vi "decodeArray.vi"(8 "error in (no error)":errorcluster, 9 "Map to Cluster?(T)":bool, 11 "ByteArray":u8[](array[numeric]) format="%x") -> (0 "error out":errorcluster, 2 "Variant":variant, 3 "RemainingBytes":u8[](array[numeric]) format="%x", 5 "Type":string)   [LabVIEW 2015, in "MsgPack.lvlib"]
uses:
  MsgPack.lvlib
panel:
  out "Array":string[](array[string])
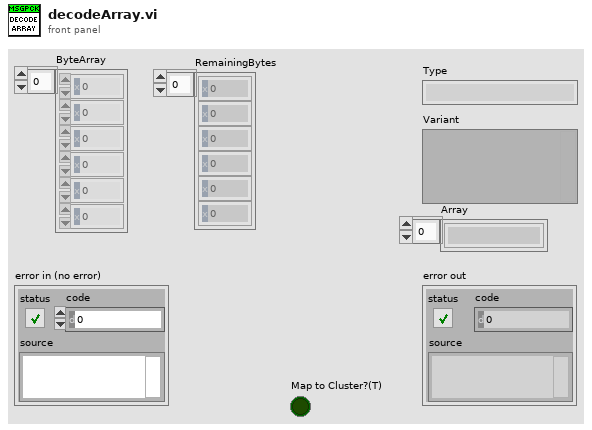
[diagram p1: front panel]
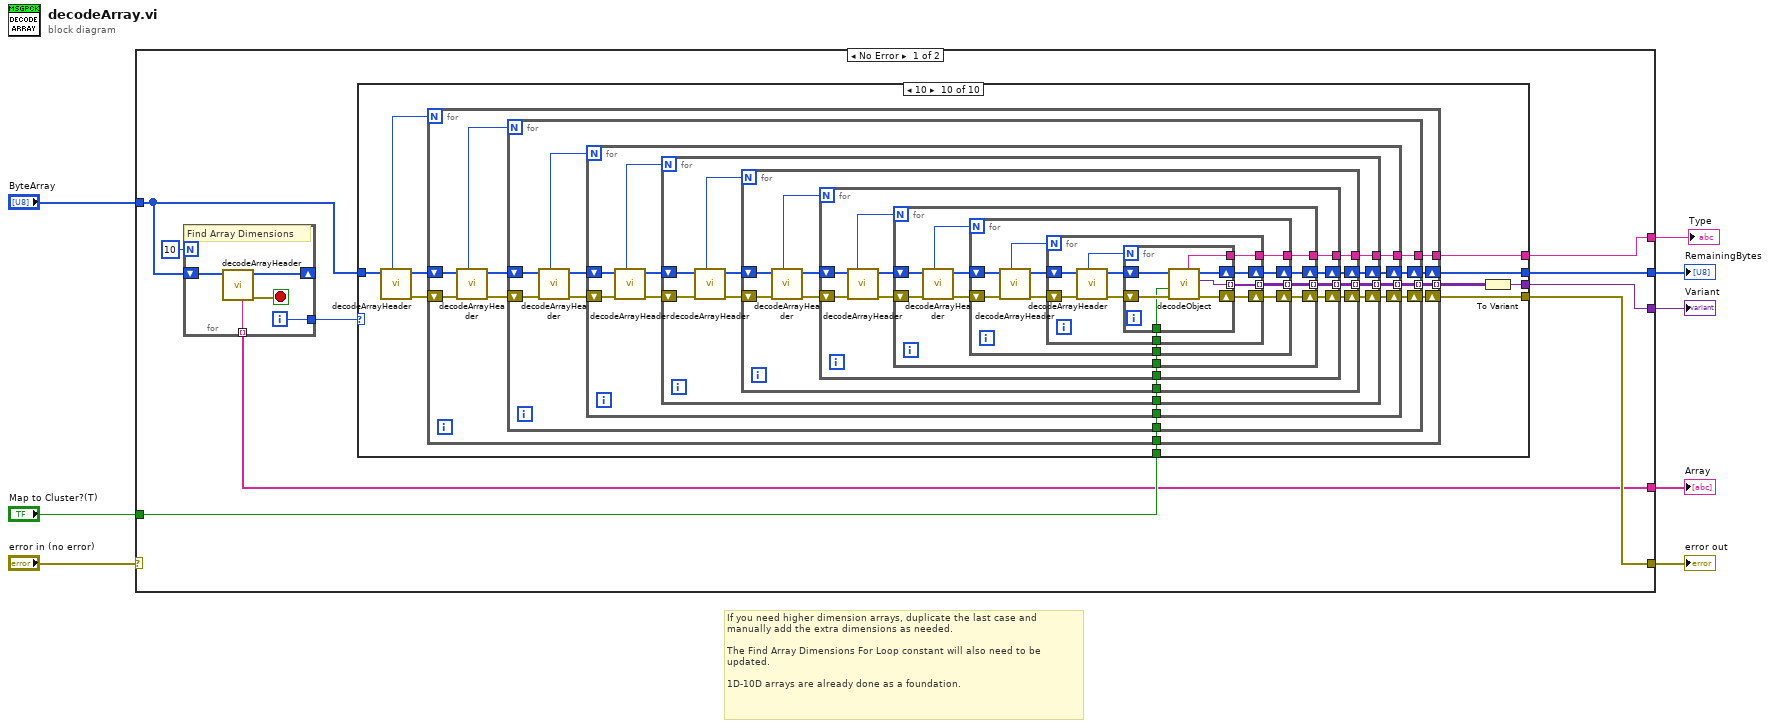
[diagram p0: block diagram]
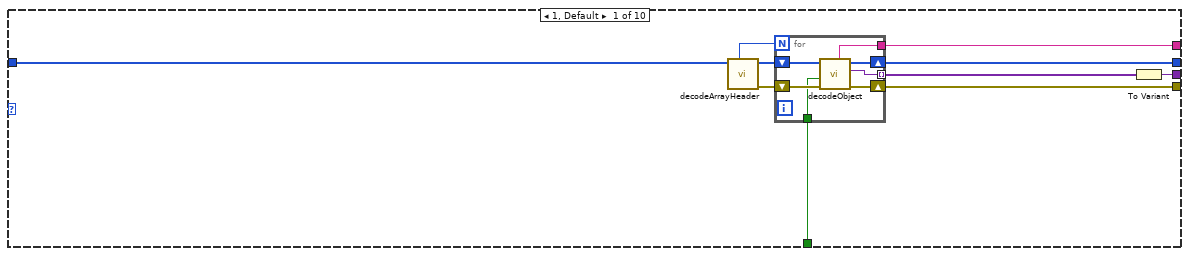
[diagram p2: hidden frame]
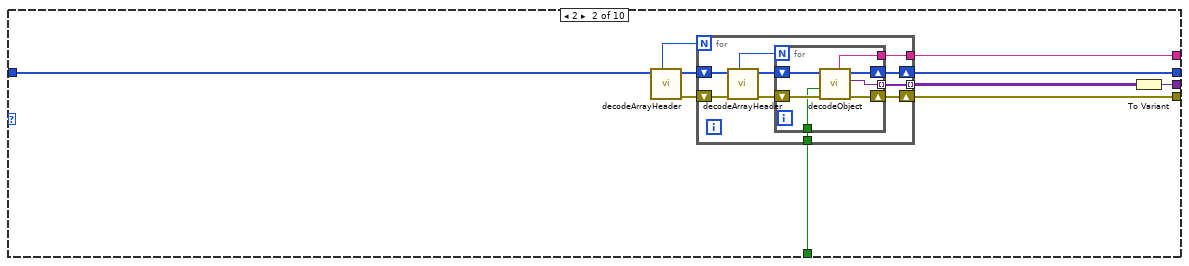
[diagram p3: hidden frame]
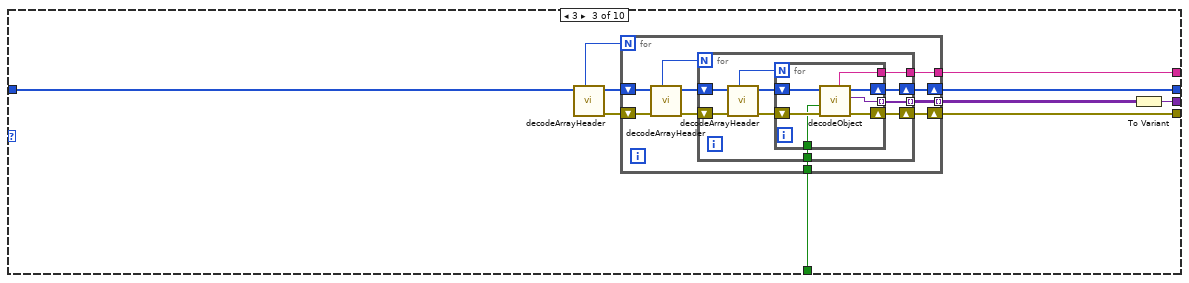
[diagram p4: hidden frame]
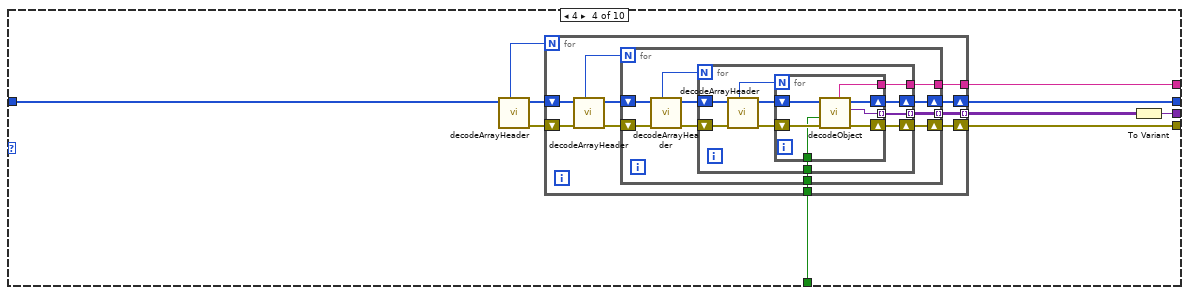
[diagram p5: hidden frame]
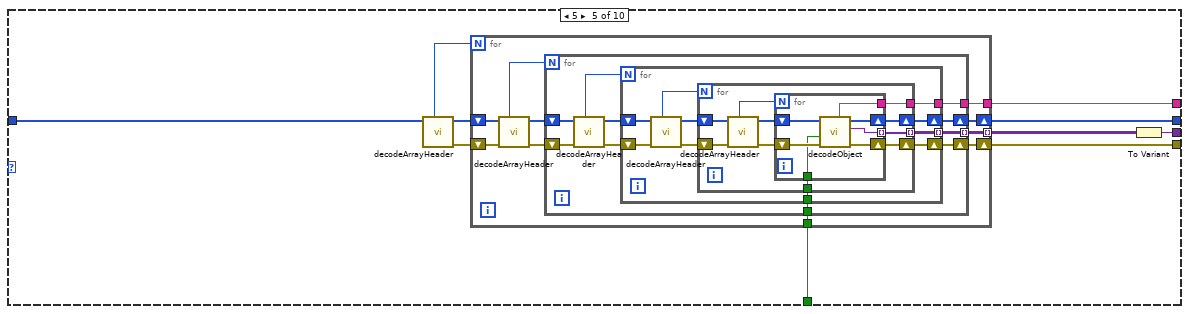
[diagram p6: hidden frame]
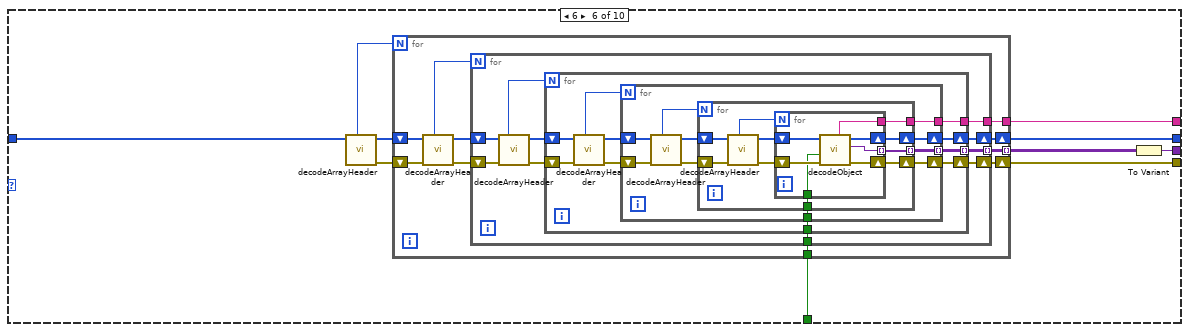
[diagram p7: hidden frame]
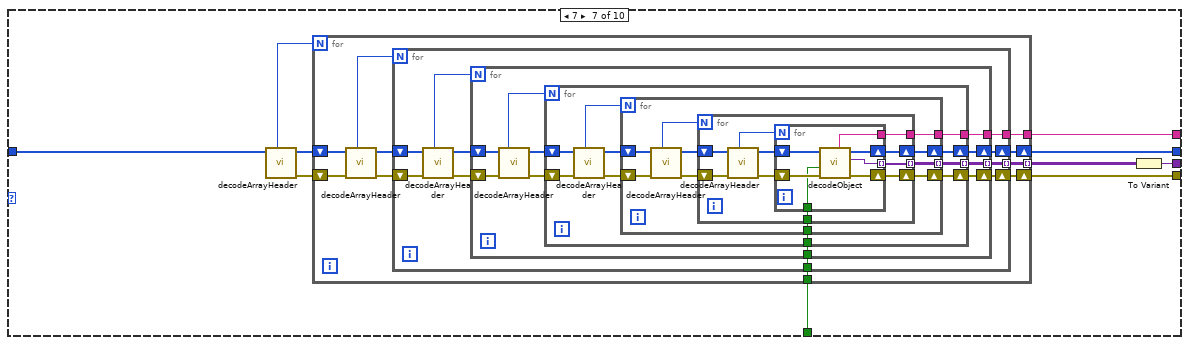
[diagram p8: hidden frame]
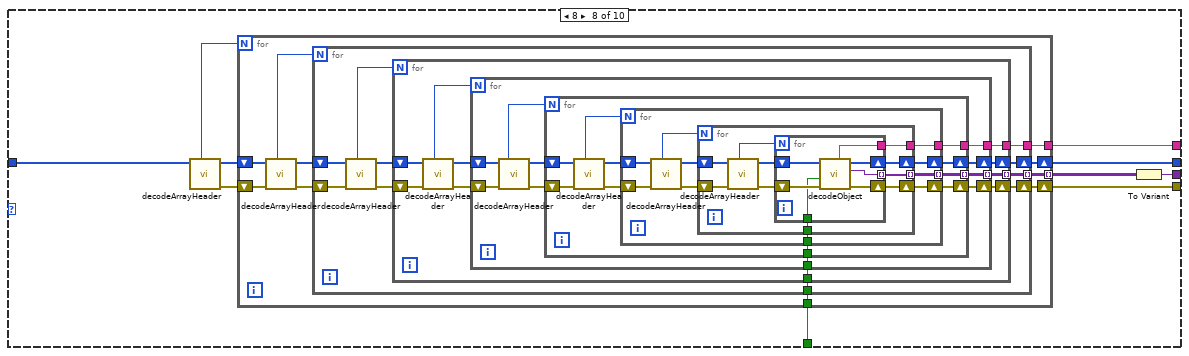
[diagram p9: hidden frame]
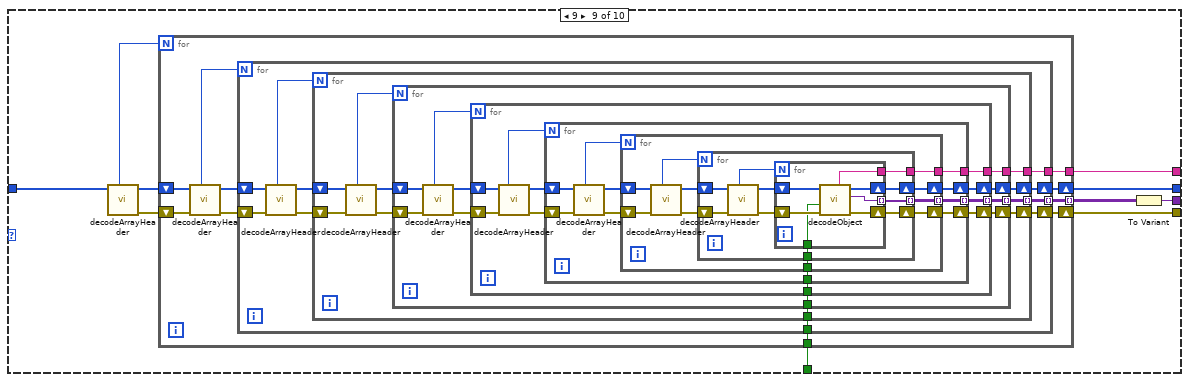
[diagram p10: hidden frame]
diagram:
  # "If you need higher dimension arrays, duplicate the last case and manually add the extra dimensions as needed.\n\nThe Find Array Dimensions For Loop constant will also need to be updated.\n\n1D-10D arrays are already done as a foundation."
  n1 = case shown="No Error" "error in (no error)" {
    selector: "error in (no error)" -> [_ w644]
    tunnel: [w17 w644] -> w8
    tunnel: "ByteArray" -> [w13 w643]
    tunnel: [w16 w643] -> w6
    tunnel: [w12 _] -> w4
    tunnel: [w11 _] -> w3
    tunnel: [w10 _] -> w2
    tunnel: "Map to Cluster?(T)" -> [w15 _]
    frame No Error {
      n2 = for {
        N: 10 -> [_]
        shift-right: [w641] -> _
        shift-left: w13 -> [w642]
        tunnel: [w639] -> w14
        tunnel: [w638] -> w11 mode=indexing
        i -> [w639]
        stop <- w640 stop-if-true
        # "Find Array Dimensions"
        n3 = call "decodeArrayHeader.vi"("ByteArray"=w642) -> ("error out"=w640:errorcluster, "RemainingBytes"=w641:u8[], "Type"=w638:string)  [unwired: 7 in, 1 out]
      }
      n4 = case shown="10" w14 {
        tunnel: [w27 w44 w71 w108 w155 w212 w279 w356 w443 w540] -> w17
        tunnel: [w26 w43 w70 w107 w154 w211 w278 w355 w442 w539] -> w16
        tunnel: w15 -> [w22 w42 w69 w106 w153 w210 w277 w354 w441 w538]
        tunnel: w13 -> [w21 w38 w65 w100 w148 w206 w271 w347 w437 w534]
        tunnel: [w19 w40 w67 w104 w151 w208 w275 w352 w439 w536] -> w12
        tunnel: [w18 w39 w66 w103 w150 w207 w274 w351 w438 w535] -> w10
        frame 1, Default {
          n5 = call "decodeArrayHeader.vi"("ByteArray"=w21) -> ("error out"=w24:errorcluster, "RemainingBytes"=w25:u8[], "Array Size"=w23:u32)  [unwired: 7 in, 1 out]
          n6 = for {
            N: w23 -> [_]
            shift-right: [w32] -> w26
            shift-left: w25 -> [w33]
            shift-right: [w30] -> w27
            shift-left: w24 -> [w34]
            tunnel: [w31] -> w20 mode=indexing
            tunnel: w22 -> [w29]
            tunnel: [w28] -> w18
            n7 = call "decodeObject.vi"("error in (no error)"=w34, "Map to Cluster?(T)"=w29, "ByteArray"=w33) -> ("error out"=w30:errorcluster, "Variant"=w31:variant, "RemainingBytes"=w32:u8[], "Type"=w28:string)  [unwired: 5 in]
          }
          n8 = To Variant(anything=w20) -> (Variant=w19:variant)
        }
        frame 2 {
          n9 = call "decodeArrayHeader.vi"("ByteArray"=w38) -> ("error out"=w36:errorcluster, "RemainingBytes"=w37:u8[], "Array Size"=w35:u32)  [unwired: 7 in, 1 out]
          n10 = for {
            N: w35 -> [_]
            tunnel: w42 -> [w49]
            tunnel: [w47] -> w41 mode=indexing
            tunnel: [w46] -> w39
            shift-right: [w53] -> w43
            shift-left: w37 -> [w48]
            shift-right: [w54] -> w44
            shift-left: w36 -> [w45]
            n11 = call "decodeArrayHeader.vi"("error in (no error)"=w45, "ByteArray"=w48) -> ("error out"=w51:errorcluster, "RemainingBytes"=w52:u8[], "Array Size"=w50:u32)  [unwired: 6 in, 1 out]
            n12 = for {
              N: w50 -> [_]
              shift-right: [w59] -> w53
              shift-left: w52 -> [w60]
              shift-right: [w57] -> w54
              shift-left: w51 -> [w61]
              tunnel: [w58] -> w47 mode=indexing
              tunnel: w49 -> [w56]
              tunnel: [w55] -> w46
              n13 = call "decodeObject.vi"("error in (no error)"=w61, "Map to Cluster?(T)"=w56, "ByteArray"=w60) -> ("error out"=w57:errorcluster, "Variant"=w58:variant, "RemainingBytes"=w59:u8[], "Type"=w55:string)  [unwired: 5 in]
            }
          }
          n14 = To Variant(anything=w41) -> (Variant=w40:variant)
        }
        frame 3 {
          n15 = call "decodeArrayHeader.vi"("ByteArray"=w65) -> ("error out"=w63:errorcluster, "RemainingBytes"=w64:u8[], "Array Size"=w62:u32)  [unwired: 7 in, 1 out]
          n16 = for {
            N: w62 -> [_]
            tunnel: w69 -> [w79]
            tunnel: [w78] -> w68 mode=indexing
            tunnel: [w77] -> w66
            shift-right: [w80] -> w70
            shift-left: w64 -> [w76]
            shift-right: [w81] -> w71
            shift-left: w63 -> [w72]
            n17 = call "decodeArrayHeader.vi"("error in (no error)"=w72, "ByteArray"=w76) -> ("error out"=w74:errorcluster, "RemainingBytes"=w75:u8[], "Array Size"=w73:u32)  [unwired: 6 in, 1 out]
            n18 = for {
              N: w73 -> [_]
              tunnel: w79 -> [w86]
              tunnel: [w84] -> w78 mode=indexing
              tunnel: [w83] -> w77
              shift-right: [w90] -> w80
              shift-left: w75 -> [w85]
              shift-right: [w91] -> w81
              shift-left: w74 -> [w82]
              n19 = call "decodeArrayHeader.vi"("error in (no error)"=w82, "ByteArray"=w85) -> ("error out"=w88:errorcluster, "RemainingBytes"=w89:u8[], "Array Size"=w87:u32)  [unwired: 6 in, 1 out]
              n20 = for {
                N: w87 -> [_]
                shift-right: [w96] -> w90
                shift-left: w89 -> [w97]
                shift-right: [w94] -> w91
                shift-left: w88 -> [w98]
                tunnel: [w95] -> w84 mode=indexing
                tunnel: w86 -> [w93]
                tunnel: [w92] -> w83
                n21 = call "decodeObject.vi"("error in (no error)"=w98, "Map to Cluster?(T)"=w93, "ByteArray"=w97) -> ("error out"=w94:errorcluster, "Variant"=w95:variant, "RemainingBytes"=w96:u8[], "Type"=w92:string)  [unwired: 5 in]
              }
            }
          }
          n22 = To Variant(anything=w68) -> (Variant=w67:variant)
        }
        frame 4 {
          n23 = call "decodeArrayHeader.vi"("ByteArray"=w100) -> ("error out"=w102:errorcluster, "RemainingBytes"=w101:u8[], "Array Size"=w99:u32)  [unwired: 7 in, 1 out]
          n24 = for {
            N: w99 -> [_]
            tunnel: w106 -> [w116]
            tunnel: [w115] -> w105 mode=indexing
            tunnel: [w114] -> w103
            shift-right: [w117] -> w107
            shift-left: w101 -> [w113]
            shift-right: [w118] -> w108
            shift-left: w102 -> [w109]
            n25 = call "decodeArrayHeader.vi"("error in (no error)"=w109, "ByteArray"=w113) -> ("error out"=w111:errorcluster, "RemainingBytes"=w112:u8[], "Array Size"=w110:u32)  [unwired: 6 in, 1 out]
            n26 = for {
              N: w110 -> [_]
              tunnel: w116 -> [w126]
              tunnel: [w125] -> w115 mode=indexing
              tunnel: [w124] -> w114
              shift-right: [w127] -> w117
              shift-left: w112 -> [w123]
              shift-right: [w128] -> w118
              shift-left: w111 -> [w119]
              n27 = call "decodeArrayHeader.vi"("error in (no error)"=w119, "ByteArray"=w123) -> ("error out"=w121:errorcluster, "RemainingBytes"=w122:u8[], "Array Size"=w120:u32)  [unwired: 6 in, 1 out]
              n28 = for {
                N: w120 -> [_]
                tunnel: w126 -> [w133]
                tunnel: [w131] -> w125 mode=indexing
                tunnel: [w130] -> w124
                shift-right: [w137] -> w127
                shift-left: w122 -> [w132]
                shift-right: [w138] -> w128
                shift-left: w121 -> [w129]
                n29 = call "decodeArrayHeader.vi"("error in (no error)"=w129, "ByteArray"=w132) -> ("error out"=w135:errorcluster, "RemainingBytes"=w136:u8[], "Array Size"=w134:u32)  [unwired: 6 in, 1 out]
                n30 = for {
                  N: w134 -> [_]
                  shift-right: [w143] -> w137
                  shift-left: w136 -> [w144]
                  shift-right: [w141] -> w138
                  shift-left: w135 -> [w145]
                  tunnel: [w142] -> w131 mode=indexing
                  tunnel: w133 -> [w140]
                  tunnel: [w139] -> w130
                  n31 = call "decodeObject.vi"("error in (no error)"=w145, "Map to Cluster?(T)"=w140, "ByteArray"=w144) -> ("error out"=w141:errorcluster, "Variant"=w142:variant, "RemainingBytes"=w143:u8[], "Type"=w139:string)  [unwired: 5 in]
                }
              }
            }
          }
          n32 = To Variant(anything=w105) -> (Variant=w104:variant)
        }
        frame 5 {
          n33 = call "decodeArrayHeader.vi"("ByteArray"=w148) -> ("error out"=w149:errorcluster, "RemainingBytes"=w147:u8[], "Array Size"=w146:u32)  [unwired: 7 in, 1 out]
          n34 = for {
            N: w146 -> [_]
            tunnel: w153 -> [w163]
            tunnel: [w162] -> w152 mode=indexing
            tunnel: [w161] -> w150
            shift-right: [w164] -> w154
            shift-left: w147 -> [w158]
            shift-right: [w165] -> w155
            shift-left: w149 -> [w157]
            n35 = call "decodeArrayHeader.vi"("error in (no error)"=w157, "ByteArray"=w158) -> ("error out"=w160:errorcluster, "RemainingBytes"=w159:u8[], "Array Size"=w156:u32)  [unwired: 6 in, 1 out]
            n36 = for {
              N: w156 -> [_]
              tunnel: w163 -> [w173]
              tunnel: [w172] -> w162 mode=indexing
              tunnel: [w171] -> w161
              shift-right: [w174] -> w164
              shift-left: w159 -> [w170]
              shift-right: [w175] -> w165
              shift-left: w160 -> [w166]
              n37 = call "decodeArrayHeader.vi"("error in (no error)"=w166, "ByteArray"=w170) -> ("error out"=w168:errorcluster, "RemainingBytes"=w169:u8[], "Array Size"=w167:u32)  [unwired: 6 in, 1 out]
              n38 = for {
                N: w167 -> [_]
                tunnel: w173 -> [w183]
                tunnel: [w182] -> w172 mode=indexing
                tunnel: [w181] -> w171
                shift-right: [w184] -> w174
                shift-left: w169 -> [w180]
                shift-right: [w185] -> w175
                shift-left: w168 -> [w176]
                n39 = call "decodeArrayHeader.vi"("error in (no error)"=w176, "ByteArray"=w180) -> ("error out"=w178:errorcluster, "RemainingBytes"=w179:u8[], "Array Size"=w177:u32)  [unwired: 6 in, 1 out]
                n40 = for {
                  N: w177 -> [_]
                  tunnel: w183 -> [w190]
                  tunnel: [w188] -> w182 mode=indexing
                  tunnel: [w187] -> w181
                  shift-right: [w194] -> w184
                  shift-left: w179 -> [w189]
                  shift-right: [w195] -> w185
                  shift-left: w178 -> [w186]
                  n41 = call "decodeArrayHeader.vi"("error in (no error)"=w186, "ByteArray"=w189) -> ("error out"=w192:errorcluster, "RemainingBytes"=w193:u8[], "Array Size"=w191:u32)  [unwired: 6 in, 1 out]
                  n42 = for {
                    N: w191 -> [_]
                    shift-right: [w200] -> w194
                    shift-left: w193 -> [w201]
                    shift-right: [w198] -> w195
                    shift-left: w192 -> [w202]
                    tunnel: [w199] -> w188 mode=indexing
                    tunnel: w190 -> [w197]
                    tunnel: [w196] -> w187
                    n43 = call "decodeObject.vi"("error in (no error)"=w202, "Map to Cluster?(T)"=w197, "ByteArray"=w201) -> ("error out"=w198:errorcluster, "Variant"=w199:variant, "RemainingBytes"=w200:u8[], "Type"=w196:string)  [unwired: 5 in]
                  }
                }
              }
            }
          }
          n44 = To Variant(anything=w152) -> (Variant=w151:variant)
        }
        frame 6 {
          n45 = call "decodeArrayHeader.vi"("ByteArray"=w206) -> ("error out"=w205:errorcluster, "RemainingBytes"=w204:u8[], "Array Size"=w203:u32)  [unwired: 7 in, 1 out]
          n46 = for {
            N: w203 -> [_]
            tunnel: w210 -> [w220]
            tunnel: [w219] -> w209 mode=indexing
            tunnel: [w218] -> w207
            shift-right: [w221] -> w211
            shift-left: w204 -> [w216]
            shift-right: [w222] -> w212
            shift-left: w205 -> [w214]
            n47 = call "decodeArrayHeader.vi"("error in (no error)"=w214, "ByteArray"=w216) -> ("error out"=w217:errorcluster, "RemainingBytes"=w215:u8[], "Array Size"=w213:u32)  [unwired: 6 in, 1 out]
            n48 = for {
              N: w213 -> [_]
              tunnel: w220 -> [w230]
              tunnel: [w229] -> w219 mode=indexing
              tunnel: [w228] -> w218
              shift-right: [w231] -> w221
              shift-left: w215 -> [w225]
              shift-right: [w232] -> w222
              shift-left: w217 -> [w224]
              n49 = call "decodeArrayHeader.vi"("error in (no error)"=w224, "ByteArray"=w225) -> ("error out"=w227:errorcluster, "RemainingBytes"=w226:u8[], "Array Size"=w223:u32)  [unwired: 6 in, 1 out]
              n50 = for {
                N: w223 -> [_]
                tunnel: w230 -> [w240]
                tunnel: [w239] -> w229 mode=indexing
                tunnel: [w238] -> w228
                shift-right: [w241] -> w231
                shift-left: w226 -> [w237]
                shift-right: [w242] -> w232
                shift-left: w227 -> [w233]
                n51 = call "decodeArrayHeader.vi"("error in (no error)"=w233, "ByteArray"=w237) -> ("error out"=w235:errorcluster, "RemainingBytes"=w236:u8[], "Array Size"=w234:u32)  [unwired: 6 in, 1 out]
                n52 = for {
                  N: w234 -> [_]
                  tunnel: w240 -> [w250]
                  tunnel: [w249] -> w239 mode=indexing
                  tunnel: [w248] -> w238
                  shift-right: [w251] -> w241
                  shift-left: w236 -> [w247]
                  shift-right: [w252] -> w242
                  shift-left: w235 -> [w243]
                  n53 = call "decodeArrayHeader.vi"("error in (no error)"=w243, "ByteArray"=w247) -> ("error out"=w245:errorcluster, "RemainingBytes"=w246:u8[], "Array Size"=w244:u32)  [unwired: 6 in, 1 out]
                  n54 = for {
                    N: w244 -> [_]
                    tunnel: w250 -> [w257]
                    tunnel: [w255] -> w249 mode=indexing
                    tunnel: [w254] -> w248
                    shift-right: [w261] -> w251
                    shift-left: w246 -> [w256]
                    shift-right: [w262] -> w252
                    shift-left: w245 -> [w253]
                    n55 = call "decodeArrayHeader.vi"("error in (no error)"=w253, "ByteArray"=w256) -> ("error out"=w259:errorcluster, "RemainingBytes"=w260:u8[], "Array Size"=w258:u32)  [unwired: 6 in, 1 out]
                    n56 = for {
                      N: w258 -> [_]
                      shift-right: [w267] -> w261
                      shift-left: w260 -> [w268]
                      shift-right: [w265] -> w262
                      shift-left: w259 -> [w269]
                      tunnel: [w266] -> w255 mode=indexing
                      tunnel: w257 -> [w264]
                      tunnel: [w263] -> w254
                      n57 = call "decodeObject.vi"("error in (no error)"=w269, "Map to Cluster?(T)"=w264, "ByteArray"=w268) -> ("error out"=w265:errorcluster, "Variant"=w266:variant, "RemainingBytes"=w267:u8[], "Type"=w263:string)  [unwired: 5 in]
                    }
                  }
                }
              }
            }
          }
          n58 = To Variant(anything=w209) -> (Variant=w208:variant)
        }
        frame 7 {
          n59 = call "decodeArrayHeader.vi"("ByteArray"=w271) -> ("error out"=w273:errorcluster, "RemainingBytes"=w272:u8[], "Array Size"=w270:u32)  [unwired: 7 in, 1 out]
          n60 = for {
            N: w270 -> [_]
            tunnel: w277 -> [w287]
            tunnel: [w286] -> w276 mode=indexing
            tunnel: [w285] -> w274
            shift-right: [w288] -> w278
            shift-left: w272 -> [w284]
            shift-right: [w289] -> w279
            shift-left: w273 -> [w280]
            n61 = call "decodeArrayHeader.vi"("error in (no error)"=w280, "ByteArray"=w284) -> ("error out"=w283:errorcluster, "RemainingBytes"=w282:u8[], "Array Size"=w281:u32)  [unwired: 6 in, 1 out]
            n62 = for {
              N: w281 -> [_]
              tunnel: w287 -> [w297]
              tunnel: [w296] -> w286 mode=indexing
              tunnel: [w295] -> w285
              shift-right: [w298] -> w288
              shift-left: w282 -> [w293]
              shift-right: [w299] -> w289
              shift-left: w283 -> [w291]
              n63 = call "decodeArrayHeader.vi"("error in (no error)"=w291, "ByteArray"=w293) -> ("error out"=w294:errorcluster, "RemainingBytes"=w292:u8[], "Array Size"=w290:u32)  [unwired: 6 in, 1 out]
              n64 = for {
                N: w290 -> [_]
                tunnel: w297 -> [w307]
                tunnel: [w306] -> w296 mode=indexing
                tunnel: [w305] -> w295
                shift-right: [w308] -> w298
                shift-left: w292 -> [w302]
                shift-right: [w309] -> w299
                shift-left: w294 -> [w301]
                n65 = call "decodeArrayHeader.vi"("error in (no error)"=w301, "ByteArray"=w302) -> ("error out"=w304:errorcluster, "RemainingBytes"=w303:u8[], "Array Size"=w300:u32)  [unwired: 6 in, 1 out]
                n66 = for {
                  N: w300 -> [_]
                  tunnel: w307 -> [w317]
                  tunnel: [w316] -> w306 mode=indexing
                  tunnel: [w315] -> w305
                  shift-right: [w318] -> w308
                  shift-left: w303 -> [w314]
                  shift-right: [w319] -> w309
                  shift-left: w304 -> [w310]
                  n67 = call "decodeArrayHeader.vi"("error in (no error)"=w310, "ByteArray"=w314) -> ("error out"=w312:errorcluster, "RemainingBytes"=w313:u8[], "Array Size"=w311:u32)  [unwired: 6 in, 1 out]
                  n68 = for {
                    N: w311 -> [_]
                    tunnel: w317 -> [w327]
                    tunnel: [w326] -> w316 mode=indexing
                    tunnel: [w325] -> w315
                    shift-right: [w328] -> w318
                    shift-left: w313 -> [w324]
                    shift-right: [w329] -> w319
                    shift-left: w312 -> [w320]
                    n69 = call "decodeArrayHeader.vi"("error in (no error)"=w320, "ByteArray"=w324) -> ("error out"=w322:errorcluster, "RemainingBytes"=w323:u8[], "Array Size"=w321:u32)  [unwired: 6 in, 1 out]
                    n70 = for {
                      N: w321 -> [_]
                      tunnel: w327 -> [w334]
                      tunnel: [w332] -> w326 mode=indexing
                      tunnel: [w331] -> w325
                      shift-right: [w338] -> w328
                      shift-left: w323 -> [w333]
                      shift-right: [w339] -> w329
                      shift-left: w322 -> [w330]
                      n71 = call "decodeArrayHeader.vi"("error in (no error)"=w330, "ByteArray"=w333) -> ("error out"=w336:errorcluster, "RemainingBytes"=w337:u8[], "Array Size"=w335:u32)  [unwired: 6 in, 1 out]
                      n72 = for {
                        N: w335 -> [_]
                        shift-right: [w344] -> w338
                        shift-left: w337 -> [w345]
                        shift-right: [w342] -> w339
                        shift-left: w336 -> [w346]
                        tunnel: [w343] -> w332 mode=indexing
                        tunnel: w334 -> [w341]
                        tunnel: [w340] -> w331
                        n73 = call "decodeObject.vi"("error in (no error)"=w346, "Map to Cluster?(T)"=w341, "ByteArray"=w345) -> ("error out"=w342:errorcluster, "Variant"=w343:variant, "RemainingBytes"=w344:u8[], "Type"=w340:string)  [unwired: 5 in]
                      }
                    }
                  }
                }
              }
            }
          }
          n74 = To Variant(anything=w276) -> (Variant=w275:variant)
        }
        frame 8 {
          n75 = call "decodeArrayHeader.vi"("ByteArray"=w347) -> ("error out"=w349:errorcluster, "RemainingBytes"=w350:u8[], "Array Size"=w348:u32)  [unwired: 7 in, 1 out]
          n76 = for {
            N: w348 -> [_]
            tunnel: w354 -> [w364]
            tunnel: [w363] -> w353 mode=indexing
            tunnel: [w362] -> w351
            shift-right: [w365] -> w355
            shift-left: w350 -> [w359]
            shift-right: [w366] -> w356
            shift-left: w349 -> [w357]
            n77 = call "decodeArrayHeader.vi"("error in (no error)"=w357, "ByteArray"=w359) -> ("error out"=w361:errorcluster, "RemainingBytes"=w360:u8[], "Array Size"=w358:u32)  [unwired: 6 in, 1 out]
            n78 = for {
              N: w358 -> [_]
              tunnel: w364 -> [w374]
              tunnel: [w373] -> w363 mode=indexing
              tunnel: [w372] -> w362
              shift-right: [w375] -> w365
              shift-left: w360 -> [w371]
              shift-right: [w376] -> w366
              shift-left: w361 -> [w367]
              n79 = call "decodeArrayHeader.vi"("error in (no error)"=w367, "ByteArray"=w371) -> ("error out"=w370:errorcluster, "RemainingBytes"=w369:u8[], "Array Size"=w368:u32)  [unwired: 6 in, 1 out]
              n80 = for {
                N: w368 -> [_]
                tunnel: w374 -> [w384]
                tunnel: [w383] -> w373 mode=indexing
                tunnel: [w382] -> w372
                shift-right: [w385] -> w375
                shift-left: w369 -> [w380]
                shift-right: [w386] -> w376
                shift-left: w370 -> [w378]
                n81 = call "decodeArrayHeader.vi"("error in (no error)"=w378, "ByteArray"=w380) -> ("error out"=w381:errorcluster, "RemainingBytes"=w379:u8[], "Array Size"=w377:u32)  [unwired: 6 in, 1 out]
                n82 = for {
                  N: w377 -> [_]
                  tunnel: w384 -> [w394]
                  tunnel: [w393] -> w383 mode=indexing
                  tunnel: [w392] -> w382
                  shift-right: [w395] -> w385
                  shift-left: w379 -> [w389]
                  shift-right: [w396] -> w386
                  shift-left: w381 -> [w388]
                  n83 = call "decodeArrayHeader.vi"("error in (no error)"=w388, "ByteArray"=w389) -> ("error out"=w391:errorcluster, "RemainingBytes"=w390:u8[], "Array Size"=w387:u32)  [unwired: 6 in, 1 out]
                  n84 = for {
                    N: w387 -> [_]
                    tunnel: w394 -> [w404]
                    tunnel: [w403] -> w393 mode=indexing
                    tunnel: [w402] -> w392
                    shift-right: [w405] -> w395
                    shift-left: w390 -> [w401]
                    shift-right: [w406] -> w396
                    shift-left: w391 -> [w397]
                    n85 = call "decodeArrayHeader.vi"("error in (no error)"=w397, "ByteArray"=w401) -> ("error out"=w399:errorcluster, "RemainingBytes"=w400:u8[], "Array Size"=w398:u32)  [unwired: 6 in, 1 out]
                    n86 = for {
                      N: w398 -> [_]
                      tunnel: w404 -> [w414]
                      tunnel: [w413] -> w403 mode=indexing
                      tunnel: [w412] -> w402
                      shift-right: [w415] -> w405
                      shift-left: w400 -> [w411]
                      shift-right: [w416] -> w406
                      shift-left: w399 -> [w407]
                      n87 = call "decodeArrayHeader.vi"("error in (no error)"=w407, "ByteArray"=w411) -> ("error out"=w409:errorcluster, "RemainingBytes"=w410:u8[], "Array Size"=w408:u32)  [unwired: 6 in, 1 out]
                      n88 = for {
                        N: w408 -> [_]
                        tunnel: w414 -> [w421]
                        tunnel: [w419] -> w413 mode=indexing
                        tunnel: [w418] -> w412
                        shift-right: [w425] -> w415
                        shift-left: w410 -> [w420]
                        shift-right: [w426] -> w416
                        shift-left: w409 -> [w417]
                        n89 = call "decodeArrayHeader.vi"("error in (no error)"=w417, "ByteArray"=w420) -> ("error out"=w423:errorcluster, "RemainingBytes"=w424:u8[], "Array Size"=w422:u32)  [unwired: 6 in, 1 out]
                        n90 = for {
                          N: w422 -> [_]
                          shift-right: [w431] -> w425
                          shift-left: w424 -> [w432]
                          shift-right: [w429] -> w426
                          shift-left: w423 -> [w433]
                          tunnel: [w430] -> w419 mode=indexing
                          tunnel: w421 -> [w428]
                          tunnel: [w427] -> w418
                          n91 = call "decodeObject.vi"("error in (no error)"=w433, "Map to Cluster?(T)"=w428, "ByteArray"=w432) -> ("error out"=w429:errorcluster, "Variant"=w430:variant, "RemainingBytes"=w431:u8[], "Type"=w427:string)  [unwired: 5 in]
                        }
                      }
                    }
                  }
                }
              }
            }
          }
          n92 = To Variant(anything=w353) -> (Variant=w352:variant)
        }
        frame 9 {
          n93 = call "decodeArrayHeader.vi"("ByteArray"=w437) -> ("error out"=w435:errorcluster, "RemainingBytes"=w436:u8[], "Array Size"=w434:u32)  [unwired: 7 in, 1 out]
          n94 = for {
            N: w434 -> [_]
            tunnel: w441 -> [w451]
            tunnel: [w450] -> w440 mode=indexing
            tunnel: [w449] -> w438
            shift-right: [w452] -> w442
            shift-left: w436 -> [w448]
            shift-right: [w453] -> w443
            shift-left: w435 -> [w444]
            n95 = call "decodeArrayHeader.vi"("error in (no error)"=w444, "ByteArray"=w448) -> ("error out"=w446:errorcluster, "RemainingBytes"=w447:u8[], "Array Size"=w445:u32)  [unwired: 6 in, 1 out]
            n96 = for {
              N: w445 -> [_]
              tunnel: w451 -> [w461]
              tunnel: [w460] -> w450 mode=indexing
              tunnel: [w459] -> w449
              shift-right: [w462] -> w452
              shift-left: w447 -> [w456]
              shift-right: [w463] -> w453
              shift-left: w446 -> [w454]
              n97 = call "decodeArrayHeader.vi"("error in (no error)"=w454, "ByteArray"=w456) -> ("error out"=w458:errorcluster, "RemainingBytes"=w457:u8[], "Array Size"=w455:u32)  [unwired: 6 in, 1 out]
              n98 = for {
                N: w455 -> [_]
                tunnel: w461 -> [w471]
                tunnel: [w470] -> w460 mode=indexing
                tunnel: [w469] -> w459
                shift-right: [w472] -> w462
                shift-left: w457 -> [w468]
                shift-right: [w473] -> w463
                shift-left: w458 -> [w464]
                n99 = call "decodeArrayHeader.vi"("error in (no error)"=w464, "ByteArray"=w468) -> ("error out"=w467:errorcluster, "RemainingBytes"=w466:u8[], "Array Size"=w465:u32)  [unwired: 6 in, 1 out]
                n100 = for {
                  N: w465 -> [_]
                  tunnel: w471 -> [w481]
                  tunnel: [w480] -> w470 mode=indexing
                  tunnel: [w479] -> w469
                  shift-right: [w482] -> w472
                  shift-left: w466 -> [w477]
                  shift-right: [w483] -> w473
                  shift-left: w467 -> [w475]
                  n101 = call "decodeArrayHeader.vi"("error in (no error)"=w475, "ByteArray"=w477) -> ("error out"=w478:errorcluster, "RemainingBytes"=w476:u8[], "Array Size"=w474:u32)  [unwired: 6 in, 1 out]
                  n102 = for {
                    N: w474 -> [_]
                    tunnel: w481 -> [w491]
                    tunnel: [w490] -> w480 mode=indexing
                    tunnel: [w489] -> w479
                    shift-right: [w492] -> w482
                    shift-left: w476 -> [w486]
                    shift-right: [w493] -> w483
                    shift-left: w478 -> [w485]
                    n103 = call "decodeArrayHeader.vi"("error in (no error)"=w485, "ByteArray"=w486) -> ("error out"=w488:errorcluster, "RemainingBytes"=w487:u8[], "Array Size"=w484:u32)  [unwired: 6 in, 1 out]
                    n104 = for {
                      N: w484 -> [_]
                      tunnel: w491 -> [w501]
                      tunnel: [w500] -> w490 mode=indexing
                      tunnel: [w499] -> w489
                      shift-right: [w502] -> w492
                      shift-left: w487 -> [w498]
                      shift-right: [w503] -> w493
                      shift-left: w488 -> [w494]
                      n105 = call "decodeArrayHeader.vi"("error in (no error)"=w494, "ByteArray"=w498) -> ("error out"=w496:errorcluster, "RemainingBytes"=w497:u8[], "Array Size"=w495:u32)  [unwired: 6 in, 1 out]
                      n106 = for {
                        N: w495 -> [_]
                        tunnel: w501 -> [w511]
                        tunnel: [w510] -> w500 mode=indexing
                        tunnel: [w509] -> w499
                        shift-right: [w512] -> w502
                        shift-left: w497 -> [w508]
                        shift-right: [w513] -> w503
                        shift-left: w496 -> [w504]
                        n107 = call "decodeArrayHeader.vi"("error in (no error)"=w504, "ByteArray"=w508) -> ("error out"=w506:errorcluster, "RemainingBytes"=w507:u8[], "Array Size"=w505:u32)  [unwired: 6 in, 1 out]
                        n108 = for {
                          N: w505 -> [_]
                          tunnel: w511 -> [w518]
                          tunnel: [w516] -> w510 mode=indexing
                          tunnel: [w515] -> w509
                          shift-right: [w522] -> w512
                          shift-left: w507 -> [w517]
                          shift-right: [w523] -> w513
                          shift-left: w506 -> [w514]
                          n109 = call "decodeArrayHeader.vi"("error in (no error)"=w514, "ByteArray"=w517) -> ("error out"=w520:errorcluster, "RemainingBytes"=w521:u8[], "Array Size"=w519:u32)  [unwired: 6 in, 1 out]
                          n110 = for {
                            N: w519 -> [_]
                            shift-right: [w528] -> w522
                            shift-left: w521 -> [w529]
                            shift-right: [w526] -> w523
                            shift-left: w520 -> [w530]
                            tunnel: [w527] -> w516 mode=indexing
                            tunnel: w518 -> [w525]
                            tunnel: [w524] -> w515
                            n111 = call "decodeObject.vi"("error in (no error)"=w530, "Map to Cluster?(T)"=w525, "ByteArray"=w529) -> ("error out"=w526:errorcluster, "Variant"=w527:variant, "RemainingBytes"=w528:u8[], "Type"=w524:string)  [unwired: 5 in]
                          }
                        }
                      }
                    }
                  }
                }
              }
            }
          }
          n112 = To Variant(anything=w440) -> (Variant=w439:variant)
        }
        frame 10 {
          n113 = call "decodeArrayHeader.vi"("ByteArray"=w534) -> ("error out"=w532:errorcluster, "RemainingBytes"=w533:u8[], "Array Size"=w531:u32)  [unwired: 7 in, 1 out]
          n114 = for {
            N: w531 -> [_]
            tunnel: w538 -> [w548]
            tunnel: [w547] -> w537 mode=indexing
            tunnel: [w546] -> w535
            shift-right: [w549] -> w539
            shift-left: w533 -> [w545]
            shift-right: [w550] -> w540
            shift-left: w532 -> [w541]
            n115 = call "decodeArrayHeader.vi"("error in (no error)"=w541, "ByteArray"=w545) -> ("error out"=w543:errorcluster, "RemainingBytes"=w544:u8[], "Array Size"=w542:u32)  [unwired: 6 in, 1 out]
            n116 = for {
              N: w542 -> [_]
              tunnel: w548 -> [w558]
              tunnel: [w557] -> w547 mode=indexing
              tunnel: [w556] -> w546
              shift-right: [w559] -> w549
              shift-left: w544 -> [w555]
              shift-right: [w560] -> w550
              shift-left: w543 -> [w551]
              n117 = call "decodeArrayHeader.vi"("error in (no error)"=w551, "ByteArray"=w555) -> ("error out"=w553:errorcluster, "RemainingBytes"=w554:u8[], "Array Size"=w552:u32)  [unwired: 6 in, 1 out]
              n118 = for {
                N: w552 -> [_]
                tunnel: w558 -> [w568]
                tunnel: [w567] -> w557 mode=indexing
                tunnel: [w566] -> w556
                shift-right: [w569] -> w559
                shift-left: w554 -> [w563]
                shift-right: [w570] -> w560
                shift-left: w553 -> [w561]
                n119 = call "decodeArrayHeader.vi"("error in (no error)"=w561, "ByteArray"=w563) -> ("error out"=w565:errorcluster, "RemainingBytes"=w564:u8[], "Array Size"=w562:u32)  [unwired: 6 in, 1 out]
                n120 = for {
                  N: w562 -> [_]
                  tunnel: w568 -> [w578]
                  tunnel: [w577] -> w567 mode=indexing
                  tunnel: [w576] -> w566
                  shift-right: [w579] -> w569
                  shift-left: w564 -> [w575]
                  shift-right: [w580] -> w570
                  shift-left: w565 -> [w571]
                  n121 = call "decodeArrayHeader.vi"("error in (no error)"=w571, "ByteArray"=w575) -> ("error out"=w574:errorcluster, "RemainingBytes"=w573:u8[], "Array Size"=w572:u32)  [unwired: 6 in, 1 out]
                  n122 = for {
                    N: w572 -> [_]
                    tunnel: w578 -> [w588]
                    tunnel: [w587] -> w577 mode=indexing
                    tunnel: [w586] -> w576
                    shift-right: [w589] -> w579
                    shift-left: w573 -> [w584]
                    shift-right: [w590] -> w580
                    shift-left: w574 -> [w582]
                    n123 = call "decodeArrayHeader.vi"("error in (no error)"=w582, "ByteArray"=w584) -> ("error out"=w585:errorcluster, "RemainingBytes"=w583:u8[], "Array Size"=w581:u32)  [unwired: 6 in, 1 out]
                    n124 = for {
                      N: w581 -> [_]
                      tunnel: w588 -> [w598]
                      tunnel: [w597] -> w587 mode=indexing
                      tunnel: [w596] -> w586
                      shift-right: [w599] -> w589
                      shift-left: w583 -> [w593]
                      shift-right: [w600] -> w590
                      shift-left: w585 -> [w592]
                      n125 = call "decodeArrayHeader.vi"("error in (no error)"=w592, "ByteArray"=w593) -> ("error out"=w595:errorcluster, "RemainingBytes"=w594:u8[], "Array Size"=w591:u32)  [unwired: 6 in, 1 out]
                      n126 = for {
                        N: w591 -> [_]
                        tunnel: w598 -> [w608]
                        tunnel: [w607] -> w597 mode=indexing
                        tunnel: [w606] -> w596
                        shift-right: [w609] -> w599
                        shift-left: w594 -> [w605]
                        shift-right: [w610] -> w600
                        shift-left: w595 -> [w601]
                        n127 = call "decodeArrayHeader.vi"("error in (no error)"=w601, "ByteArray"=w605) -> ("error out"=w603:errorcluster, "RemainingBytes"=w604:u8[], "Array Size"=w602:u32)  [unwired: 6 in, 1 out]
                        n128 = for {
                          N: w602 -> [_]
                          tunnel: w608 -> [w618]
                          tunnel: [w617] -> w607 mode=indexing
                          tunnel: [w616] -> w606
                          shift-right: [w619] -> w609
                          shift-left: w604 -> [w615]
                          shift-right: [w620] -> w610
                          shift-left: w603 -> [w611]
                          n129 = call "decodeArrayHeader.vi"("error in (no error)"=w611, "ByteArray"=w615) -> ("error out"=w613:errorcluster, "RemainingBytes"=w614:u8[], "Array Size"=w612:u32)  [unwired: 6 in, 1 out]
                          n130 = for {
                            N: w612 -> [_]
                            tunnel: w618 -> [w625]
                            tunnel: [w623] -> w617 mode=indexing
                            tunnel: [w622] -> w616
                            shift-right: [w629] -> w619
                            shift-left: w614 -> [w624]
                            shift-right: [w630] -> w620
                            shift-left: w613 -> [w621]
                            n131 = call "decodeArrayHeader.vi"("error in (no error)"=w621, "ByteArray"=w624) -> ("error out"=w627:errorcluster, "RemainingBytes"=w628:u8[], "Array Size"=w626:u32)  [unwired: 6 in, 1 out]
                            n132 = for {
                              N: w626 -> [_]
                              shift-right: [w635] -> w629
                              shift-left: w628 -> [w636]
                              shift-right: [w633] -> w630
                              shift-left: w627 -> [w637]
                              tunnel: [w634] -> w623 mode=indexing
                              tunnel: w625 -> [w632]
                              tunnel: [w631] -> w622
                              n133 = call "decodeObject.vi"("error in (no error)"=w637, "Map to Cluster?(T)"=w632, "ByteArray"=w636) -> ("error out"=w633:errorcluster, "Variant"=w634:variant, "RemainingBytes"=w635:u8[], "Type"=w631:string)  [unwired: 5 in]
                            }
                          }
                        }
                      }
                    }
                  }
                }
              }
            }
          }
          n134 = To Variant(anything=w537) -> (Variant=w536:variant)
        }
      }
    }
    frame Error {
    }
  }
  "error out" <- w8
  "Variant" <- w4
  "Type" <- w2
  "RemainingBytes" <- w6
  "Array" <- w3
